vi "SubVITemp.vi"(11 "°F":dbl) -> (3 "Numeric":dbl)   [LabVIEW 2021]
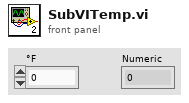
[diagram p1: front panel]
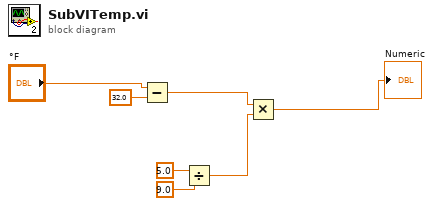
[diagram p0: block diagram]
diagram:
  n1 = Subtract(x="°F", y=32.0) -> (x-y=w5:dbl)
  n2 = Divide(x=5.0, y=9.0) -> (x/y=w6:dbl)
  n3 = Multiply(x=w5, y=w6) -> (x*y=→"Numeric":dbl)
